vi "Complex Generalized SVD Decomposition.vi"(0 "A":T2, 5 "B":T2, 7 "singular values only?":bool, 9 "SVD option":T3 items=["Thin", "Full"]) -> (3 "Singular Values":dbl[](array[numeric]), 4 "Matrix U":T2, 6 "Matrix V":T2, 8 "Matrix C":T1, 10 "Matrix S":T1, 14 "Matrix R":T2, 15 "error":i32)   [LabVIEW 2017, in "NI_AALPro.lvlib"]
doc: "Computes the generalized singular value decomposition (GSVD) of a matrix pair (<B>A</B>,<B>B</B>). The data types you wire to the <B>A</B> and <B>B</B> inputs determine the polymorphic instance to use."
uses:
  <vilib>/Analysis/NI_AALPro.lvlib
  <vilib>/Analysis/Matrix/Datatypes/ComplexMatrix.ctl
  <vilib>/Analysis/7linalg.llb/SVD Option.ctl
  <vilib>/Analysis/Matrix/Datatypes/RealMatrix.ctl
  <resource>/lvanlys.dll
  <vilib>/Analysis/Matrix/NI_Matrix.lvlib
panel:
  # "Generalized SVD Decomposition"
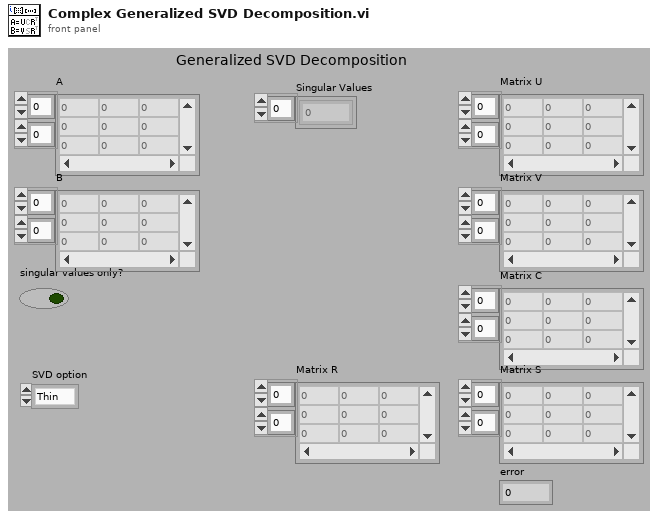
[diagram p1: front panel]
types:
  T1 = typedef "NI_Matrix.lvlib/RealMatrix.ctl" = dbl[][]
  T2 = typedef "NI_Matrix.lvlib/ComplexMatrix.ctl" = cdb[][]
  T3 = typedef "NI_AALPro.lvlib/SVD Option.ctl" = u16
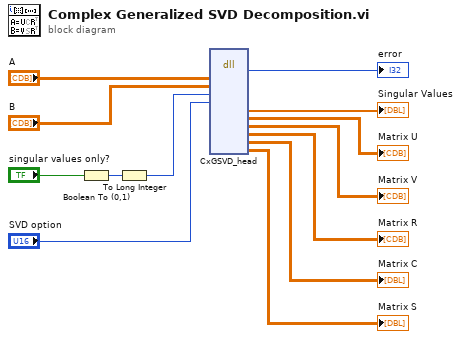
[diagram p0: block diagram]
diagram:
  n1 = Boolean To (0,1)(Boolean="singular values only?") -> (0, 1=w7:i16)
  n2 = To Long Integer(number=w7) -> (32bit integer=w6:i32)
  n3 = dll-call lib="e:/builds/penguin/labview/branches/2017/dev/dist/resource/lvanlys.*" fn="CxGSVD_head"("aH"="A", "bH"="B", "job"=w6, "opt"="SVD option") -> ("return type"=→"error":i32, "sval"=→"Singular Values":dbl[], "Matrix U"=→"Matrix U":T2, "Matrix V"=→"Matrix V":T2, "Matrix R"=→"Matrix R":T2, "cH"=→"Matrix C":dbl[][], "sH"=→"Matrix S":dbl[][])  [unwired: 13 in, 2 out]
